vi "GlobalRegEd.vi"(4 "params":u8[](array[numeric])=[32, 22]) -> (1 "Global Reg out":u32[](array[numeric]) format="%.0x")   [LabVIEW 2015, in "VIPM2.lvlib"]
doc: "params:\n Analog Vref low (ring)\n Gb THLD (ring)"
uses:
  VIPM2.lvlib
panel:
  # "Analog Vref low"
  # "Gb THLD"
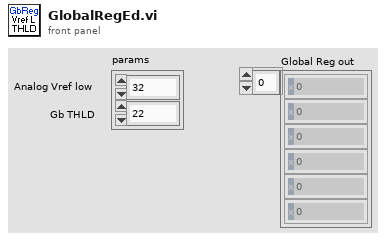
[diagram p1: front panel]
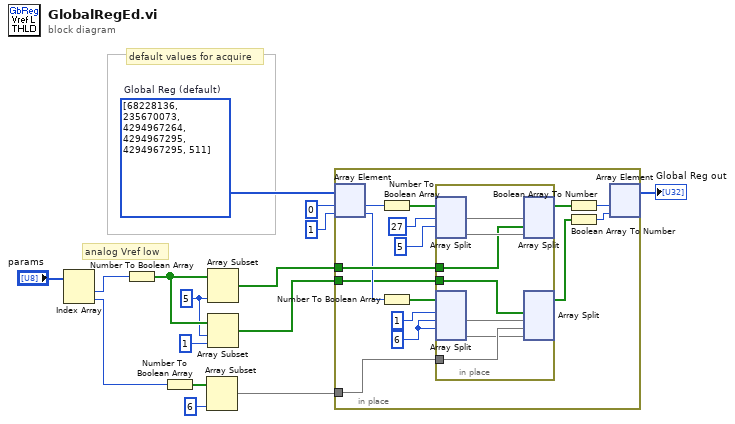
[diagram p0: block diagram]
diagram:
  w5 = 5 ("length")
  w15 = u32[] [68228136, 235670073, 4294967264, 4294967295, 4294967295, 511]  # Global Reg (default)
  # "analog Vref low"
  # "default values for acquire"
  n1 = Index Array(array="params") -> (element #1=w7:u8, element #2=w1:u8)  [unwired: 2 in]
  n2 = Number To Boolean Array(number=w7) -> (Boolean array=w6:bool[])
  n3 = Number To Boolean Array(number=w1) -> (Boolean array=w9:bool[])
  n4 = Array Subset "Array Subset"(array=w9, length=6) -> (w8:bool[])  [unwired: 1 in]
  n5 = Array Subset "Array Subset"(array=w6, length=w5) -> (w13:bool[])  [unwired: 1 in]
  n6 = Array Subset(array=w6, index=w5, length=1) -> (w3:bool[])
  n7 = in-place {
    in-place-border: w13 -> [w26]
    in-place-border: w8 -> [w19]
    in-place-border: w3 -> [w21]
    w20 = 6
    n8 = in-place-array #1(w15, 0, 1) -> (w30:u32, w24:u32)
    n9 = Number To Boolean Array(number=w30) -> (Boolean array=w29:bool[])
    n10 = Number To Boolean Array(number=w24) -> (Boolean array=w23:bool[])
    n11 = in-place {
      in-place-border: w26 -> [w35]
      in-place-border: w21 -> [w34]
      in-place-border: w19 -> [w32]
      n12 = in-place-split #2(w29, 27, 5) -> (w37:bool[], w36:bool[])  [unwired: 1 out]
      n13 = in-place-split #3(w23, 1, w20, w20) -> (w33:bool[], w31:bool[])  [unwired: 2 out]
      n14 = in-place-split #2(w37, w35, w36) -> (w18:bool[])  [unwired: 2 out]
      n15 = in-place-split #3(w34, w33, w32, w31) -> (w17:bool[])  [unwired: 3 out]
    }
    n16 = Boolean Array To Number(Boolean array=w18) -> (number=w25:u32)
    n17 = Boolean Array To Number(Boolean array=w17) -> (number=w16:u32)
    n18 = in-place-array #1(w25, w16) -> (→"Global Reg out":u32[])  [unwired: 2 out]
  }
